vi "Config PWM.vi"(8 "error in (no error)":errorcluster, 11 "Data":variant) -> (0 "error out":errorcluster)   [LabVIEW 2023, in "FPGA.lvlib"]
uses:
  FPGA.lvlib
  Internal Communication/Controls/Queue.ctl
panel:
  out "Queue Out":T1
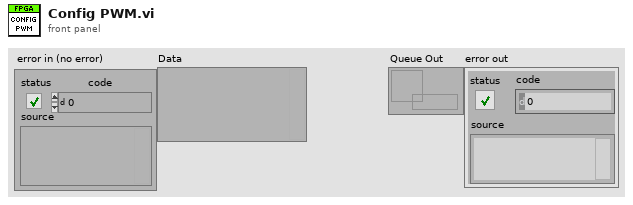
[diagram p1: front panel]
types:
  T1 = typedef "Queue.ctl" = refnum<queue>
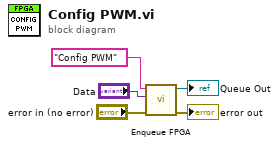
[diagram p0: block diagram]
diagram:
  n1 = call "Enqueue FPGA.vi"("error in (no error)"="error in (no error)", "Data"="Data", "Command"="Config PWM") -> ("error out"=→"error out":errorcluster, "Queue Out"=→"Queue Out":T1)  [unwired: 7 in]
